vi "TTA_MATLAB_Tile_Set_PA_PowerMeas_Cal.vi"(0 "Channels":string[](array[combo]), 1 "Frequency":dbl, 5 "Index":i32, 7 "Power":dbl, 11 "error in":errorcluster) -> (4 "Success":bool, 6 "TileSuccessComm":bool[](array[boolean]), 8 "TileSuccessOp":bool[](array[boolean]), 10 "Tile Outputs":dbl[][](array[numeric]), 15 "error out":errorcluster)   [LabVIEW 2016]
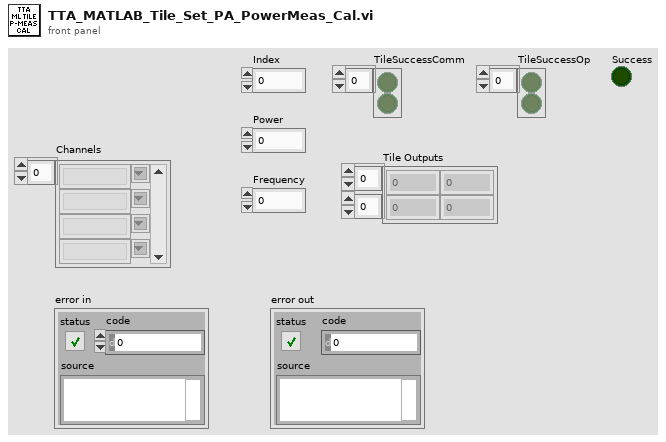
[diagram p1: front panel]
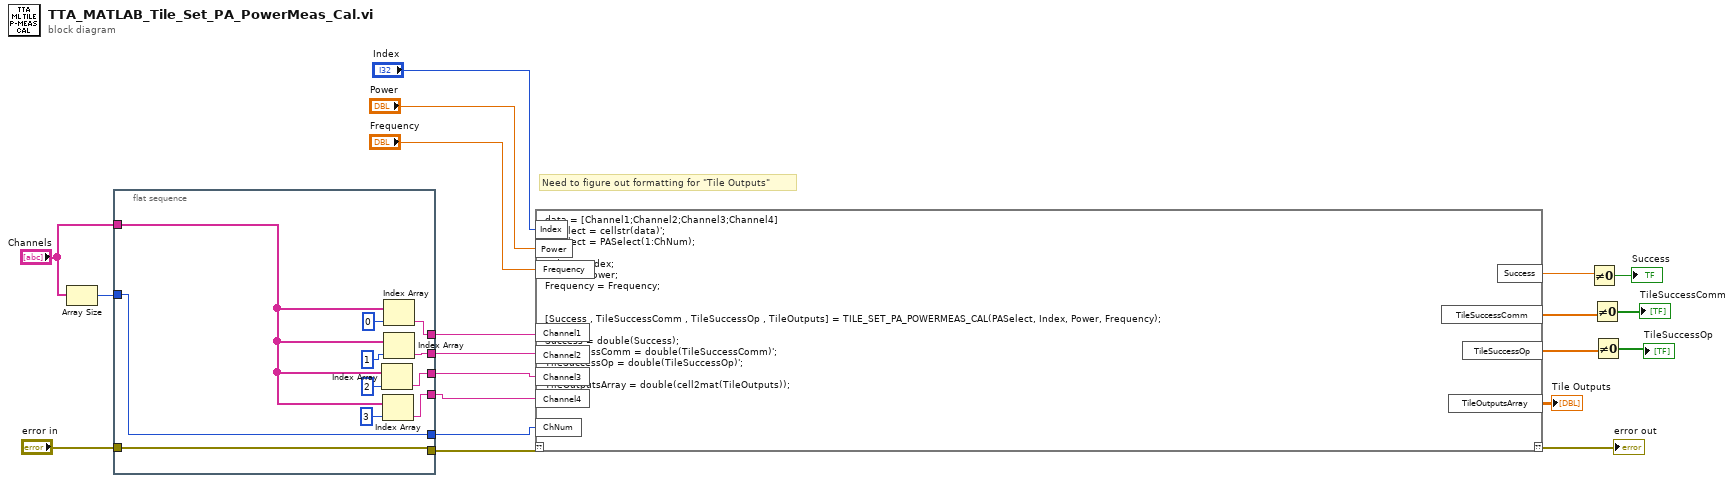
[diagram p0: block diagram]
diagram:
  # "Need to figure out formatting for \"Tile Outputs\""
  n1 = Array Size(array="Channels") -> (size(s)=w11:i32)
  n2 = flat-sequence {
    tunnel: "error in" -> [w31]
    tunnel: [w30] -> w7
    tunnel: w11 -> [w24]
    tunnel: [w31] -> w8
    tunnel: "Channels" -> [w23]
    tunnel: [w27] -> w5
    tunnel: [w25] -> w4
    tunnel: [w24] -> w6
    tunnel: [w21] -> w3
    frame #0 {
      n3 = Index Array(array=w23, index=2) -> (element=w25:string)
      n4 = Index Array(array=w23, index=3) -> (element=w21:string)
      n5 = Index Array(array=w23, index=0) -> (element=w30:string)
      n6 = Index Array(array=w23, index=1) -> (element=w27:string)
    }
  }
  n7 = script code="data = [Channel1;Channel2;Channel3;Channel4]\nPASelect = cellstr(data)';\nPASelect = PASelect(1:ChNum);\n\nIndex = Index;\nPower = Power;\nFrequency = Frequency;\n\n\n[Success , TileSuccessComm , TileSuccessOp , TileOutputs] = TILE_SET_PA_POWERMEAS_CAL(PASelect, Index, Power, Frequency);\n\nSuccess = double(Success);\nTileSuccessComm = double(TileSuccessComm)';\nTileSuccessOp = double(TileSuccessOp)';\n\nTileOutputsArray = double(cell2mat(TileOutputs));"("??"=w8, "Channel1"=w7, "Index"="Index", "Power"="Power", "Frequency"="Frequency", "Channel2"=w5, "Channel3"=w4, "Channel4"=w3, "ChNum"=w6) -> ("??"=→"error out":errorcluster, "Success"=w14:dbl, "TileSuccessComm"=w13:dbl[], "TileSuccessOp"=w12:dbl[], "TileOutputsArray"=→"Tile Outputs":dbl[][])
  n8 = Not Equal To 0?(x=w14) -> (x != 0?=→"Success":bool)
  n9 = Not Equal To 0?(x=w13) -> (x != 0?=→"TileSuccessComm":bool[])
  n10 = Not Equal To 0?(x=w12) -> (x != 0?=→"TileSuccessOp":bool[])
